vi "Frame Sync In.vi"(5 "format (sample clock)":T1(ring), 6 "channel count (2)":u8=2, 7 "data sample edge (rising)":enum16{"rising", "falling"}(ring), 8 "receive":bool, 9 "prev output valid":bool, 10 "frame sync in":bool, 11 "clock in":bool) -> (0 "latch config":bool, 1 "force output":bool, 2 "start read":bool)   [LabVIEW 2013, in "I2S-TDM.lvlib"]
uses:
  I2S-TDM.lvlib
  Controls/tdm transmit states.ctl
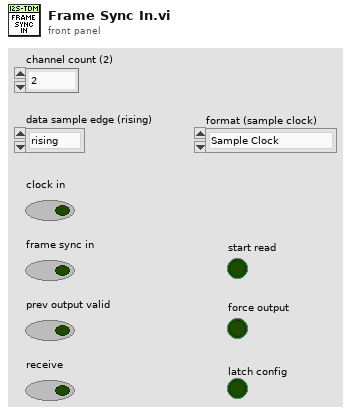
[diagram p1: front panel]
types:
  T1 = enum16{"Sample Clock", "Pre-Start Pulse", "Word Select (I2S only)"}
  T2 = typedef "I2S-TDM.lvlib/tdm transmit states.ctl" = enum16{"idle", "pre-transfer", "transfer"}
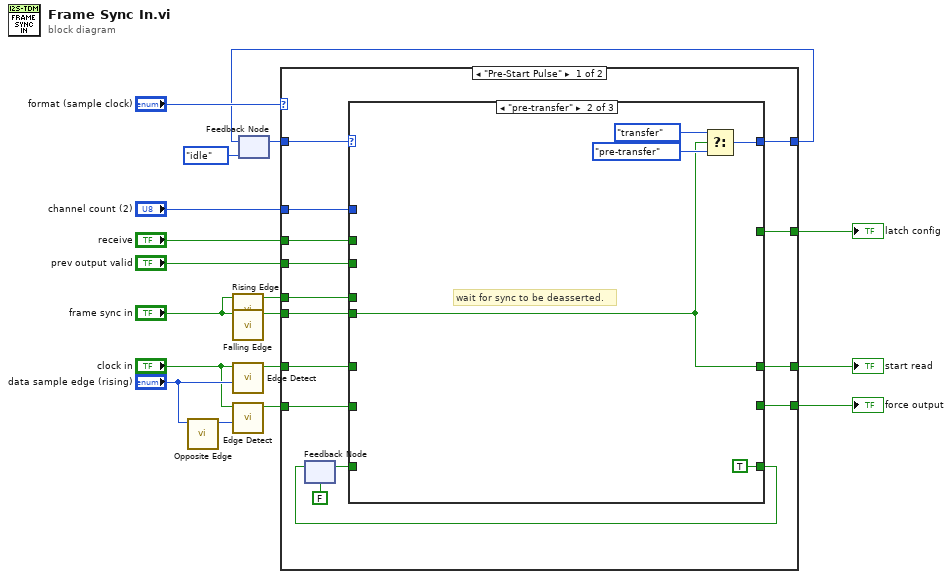
[diagram p0: block diagram]
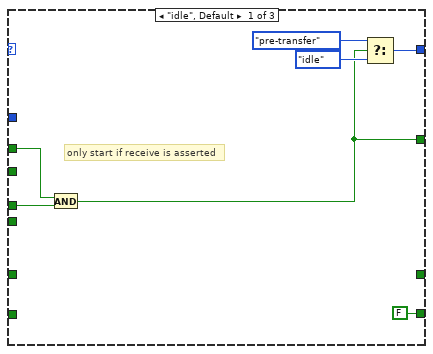
[diagram p2: hidden frame]
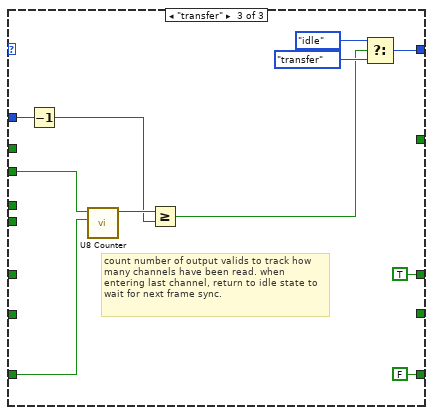
[diagram p3: hidden frame]
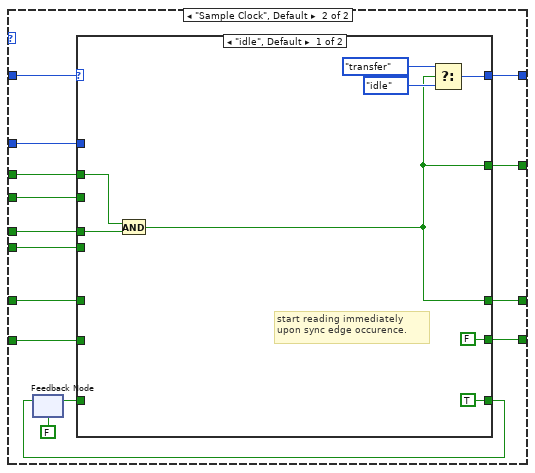
[diagram p4: hidden frame]
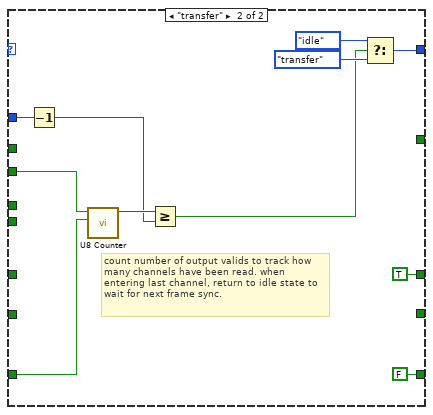
[diagram p5: hidden frame]
diagram:
  n1 = call "Opposite Edge.vi"("edge in"="data sample edge (rising)") -> ("opposite edge out"=w7:enum16{"rising", "falling"})  [unwired: 10 in]
  n2 = call "Rising Edge.vi"("signal in"="frame sync in") -> ("rising edge?"=w3:bool)  [unwired: 10 in]
  n3 = call "Falling Edge.vi"("signal in"="frame sync in") -> ("falling edge?"=w2:bool)  [unwired: 10 in]
  n4 = call "Edge Detect.vi"("edge (rising)"="data sample edge (rising)", "signal in"="clock in") -> ("edge detected?"=w16:bool)  [unwired: 9 in]
  n5 = call "Edge Detect.vi"("edge (rising)"=w7, "signal in"="clock in") -> ("edge detected?"=w5:bool)  [unwired: 9 in]
  n6 = feedback #1(tdm_transmit_states."idle") -> (w17:T2)
  n7 = case shown="\"Pre-Start Pulse\"" "format (sample clock)" {
    tunnel: w17 -> [w33 w71]
    tunnel: [w32 w70] -> w12
    tunnel: w16 -> [w31 w69]
    tunnel: "receive" -> [w30 w68]
    tunnel: "channel count (2)" -> [w29 w67]
    tunnel: w2 -> [w20 w58]
    tunnel: [w28 w66] -> w11
    tunnel: [w27 w65] -> w10
    tunnel: [w26 w64] -> w9
    tunnel: w5 -> [w25 w63]
    tunnel: "prev output valid" -> [w23 w61]
    tunnel: w3 -> [w19 w57]
    frame "Pre-Start Pulse" {
      n8 = feedback #2(FALSE) -> (w24:bool)
      n9 = case shown="\"pre-transfer\"" w33 {
        tunnel: [w38 w43 w47] -> w32
        tunnel: w30 -> [w36 _ _]
        tunnel: w31 -> [_ _ _]
        tunnel: [_ w41 TRUE ("edge detected?")] -> w27
        tunnel: w29 -> [_ _ w55]
        tunnel: w20 -> [_ w41 _]
        tunnel: w19 -> [w37 _ _]
        tunnel: [w34 _ _] -> w28
        tunnel: [FALSE ("latched signal") _ _] -> w26
        tunnel: w25 -> [_ _ _]
        tunnel: [_ TRUE FALSE] -> w22
        tunnel: w24 -> [_ _ w54]
        tunnel: w23 -> [_ _ w53]
        frame "idle", Default {
          # "only start if receive is asserted"
          n10 = And(x=w36, y=w37) -> (x .and. y?=w34:bool)
          n11 = Select(t=tdm_transmit_states."pre-transfer", s=w34, f=tdm_transmit_states."idle") -> (s? t:f=w38:T2)
        }
        frame "pre-transfer" {
          # "wait for sync to be deasserted."
          n12 = Select(t=tdm_transmit_states."transfer", s=w41, f=tdm_transmit_states."pre-transfer") -> (s? t:f=w43:T2)
        }
        frame "transfer" {
          # "count number of output valids to track how many channels have been read. when entering last channel, return to idle state to wait for next frame sync."
          n13 = Decrement(x=w55) -> (x-1=w50:u8)
          n14 = call "U8 Counter.vi"("reset (F)"=w54, "increment"=w53) -> ("count"=w51:u8)  [unwired: 9 in]
          n15 = Greater Or Equal?(x=w51, y=w50) -> (x >= y?=w46:bool)
          n16 = Select(t=tdm_transmit_states."idle", s=w46, f=tdm_transmit_states."transfer") -> (s? t:f=w47:T2)
        }
      }
      n17 = feedback-in #2(w22) -> ()
    }
    frame "Sample Clock", Default {
      n18 = feedback #3(FALSE) -> (w62:bool)
      n19 = case shown="\"idle\", Default" w71 {
        tunnel: [w77 w82] -> w70
        tunnel: w68 -> [w75 _]
        tunnel: w69 -> [_ _]
        tunnel: [w73 TRUE ("edge detected?")] -> w65
        tunnel: w67 -> [_ w89]
        tunnel: w58 -> [_ _]
        tunnel: w57 -> [w76 _]
        tunnel: [w73 _] -> w66
        tunnel: [FALSE ("latched signal") _] -> w64
        tunnel: w63 -> [_ _]
        tunnel: [TRUE FALSE] -> w60
        tunnel: w62 -> [_ w88]
        tunnel: w61 -> [_ w87]
        frame "idle", Default {
          # "start reading immediately upon sync edge occurence."
          n20 = And(x=w75, y=w76) -> (x .and. y?=w73:bool)
          n21 = Select(t=tdm_transmit_states."transfer", s=w73, f=tdm_transmit_states."idle") -> (s? t:f=w77:T2)
        }
        frame "transfer" {
          # "count number of output valids to track how many channels have been read. when entering last channel, return to idle state to wait for next frame sync."
          n22 = Decrement(x=w89) -> (x-1=w80:u8)
          n23 = call "U8 Counter.vi"("reset (F)"=w88, "increment"=w87) -> ("count"=w85:u8)  [unwired: 9 in]
          n24 = Greater Or Equal?(x=w85, y=w80) -> (x >= y?=w81:bool)
          n25 = Select(t=tdm_transmit_states."idle", s=w81, f=tdm_transmit_states."transfer") -> (s? t:f=w82:T2)
        }
      }
      n26 = feedback-in #3(w60) -> ()
    }
  }
  "start read" <- w10
  "latch config" <- w11
  "force output" <- w9
  n27 = feedback-in #1(w12) -> ()
